vi "Read Main VI.vi"(8 "error in (no error)":errorcluster, 11 "Tax_calculation in":refnum<class "Tax_calculation.lvclass">) -> (0 "error out":errorcluster, 2 "Main VI":refnum<vi>, 3 "Tax_calculation out":refnum<class "Tax_calculation.lvclass">)   [LabVIEW 2016, in "Tax_calculation.lvclass"]
uses:
  Tax_calculation.lvclass
  Tax_calculation.lvclass/Tax_calculation.ctl
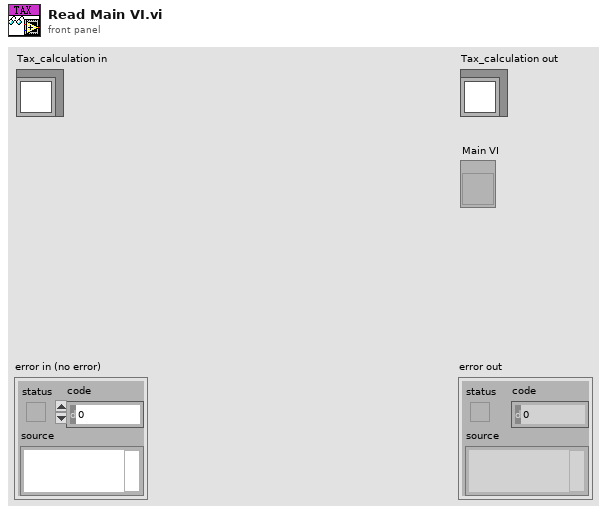
[diagram p1: front panel]
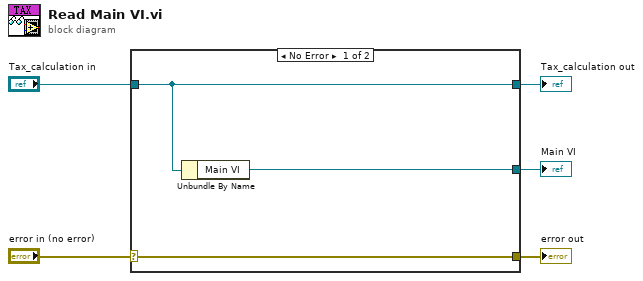
[diagram p0: block diagram]
diagram:
  n1 = case shown="No Error" "error in (no error)" {
    selector: "error in (no error)" -> [w8 w9]
    tunnel: [w8 w9] -> w4
    tunnel: [w7 w10] -> w2
    tunnel: "Tax_calculation in" -> [w7 w10]
    tunnel: [w6 _] -> w1
    frame No Error {
      n2 = Unbundle By Name(w7) -> ("Main VI"=w6:refnum<vi>)
    }
    frame Error {
    }
  }
  "error out" <- w4
  "Tax_calculation out" <- w2
  "Main VI" <- w1
